vi "User Config Write Value.vi"(7 "Section":string, 8 "error in (no error)":errorcluster, 9 "Value":string, 10 "Key":string, 11 "INI File Path":path) -> (0 "error out":errorcluster, 2 "overwritten?":bool, 3 "INI File Path":path)   [LabVIEW 2024]
uses:
  <vilib>/Utility/config.llb/NI_LVConfig.lvlib
  <vilib>/Utility/config.llb/Write Key (String).vi
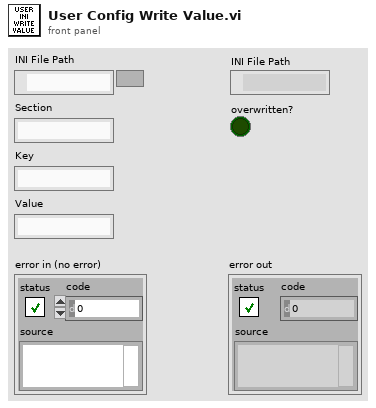
[diagram p1: front panel]
types:
  T1 = typedef "NI_LVConfig.lvlib/Config Data RefNum.ctl" = refnum<k1>
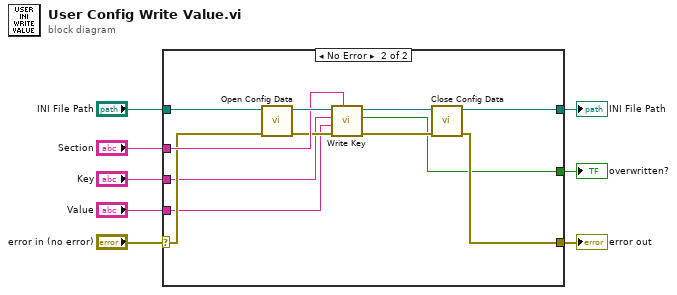
[diagram p0: block diagram]
diagram:
  n1 = case shown="No Error" "error in (no error)" {
    selector: "error in (no error)" -> [w9 w18]
    tunnel: [w9 w12] -> w7
    tunnel: "INI File Path" -> [_ w21]
    tunnel: "Section" -> [_ w19]
    tunnel: "Key" -> [_ w16]
    tunnel: "Value" -> [_ w15]
    tunnel: [_ w11] -> w2
    tunnel: [_ w10] -> w1
    frame Error {
    }
    frame No Error {
      n2 = call <vilib>:"Open Config Data.vi"("error in (no error)"=w18, "configuration file path"=w21) -> ("error out"=w17:errorcluster, "refnum"=w20:T1)  [unwired: 7 in, 1 out]
      n3 = call-poly <vilib>:"Write Key.vi"("section"=w19, "error in (no error)"=w17, "value"=w15, "key"=w16, "refnum"=w20) -> ("error out"=w13:errorcluster, "found?"=w10:bool, "refnum out"=w14:T1)  [unwired: 4 in]
      n4 = call <vilib>:"Close Config Data.vi"("error in (no error)"=w13, "refnum"=w14) -> ("error out"=w12:errorcluster, "file path"=w11:path)  [unwired: 8 in]
    }
  }
  "error out" <- w7
  "INI File Path" <- w2
  "overwritten?" <- w1
